vi "sv_Check for Bandwidth Change.vi"(7 "reset filter (F)":bool, 8 "error in (no error)":errorcluster, 9 "1/n octave settings":T2) -> (0 "error out":errorcluster, 1 "bandwidth":T3(ring), 2 "parameter has changed":bool)   [LabVIEW 2017, in "SoundVib_Octave_2014 standard.lvlib"]
uses:
  <vilib>/addons/Sound and Vibration/svt_Octave/SoundVib_Octave_2014 standard.lvlib
  <vilib>/addons/_NISVFA/_Shared subVIs/Controls/svc_Octave Standard.ctl
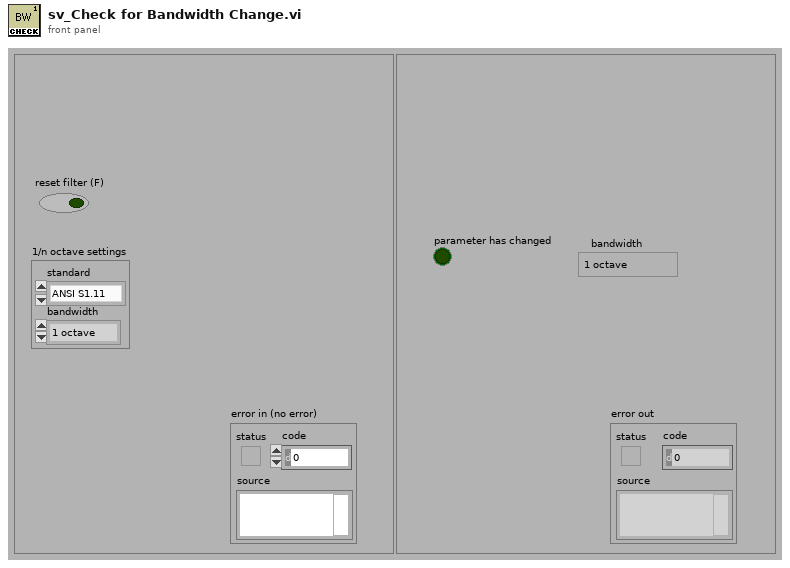
[diagram p1: front panel]
types:
  T1 = typedef "svc_Octave Standard.ctl" = enum16{"ANSI S1.11", "IEC 61260"}
  T2 = cluster{"standard":T1, "bandwidth":enum16{"1 octave", "1/3 octave", "1/6 octave", "1/12 octave", "1/24 octave"}}
  T3 = enum16{"1 octave", "1/3 octave", "1/6 octave", "1/12 octave", "1/24 octave"}
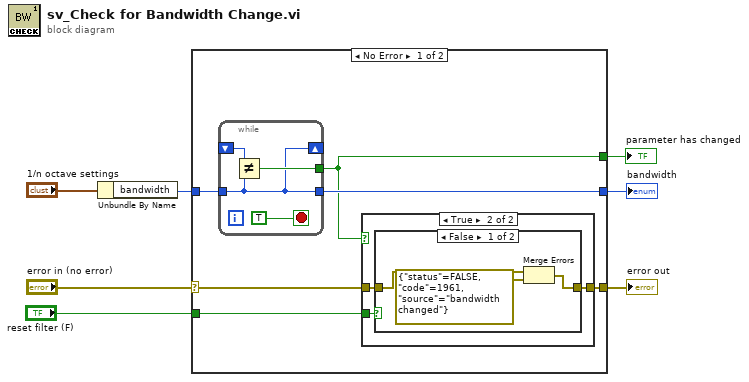
[diagram p0: block diagram]
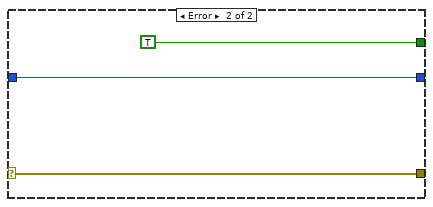
[diagram p4: hidden frame]
diagram:
  n1 = Unbundle By Name("1/n octave settings") -> ("bandwidth"=w4:T3)
  n2 = case shown="No Error" "error in (no error)" {
    selector: "error in (no error)" -> [w10 w28]
    tunnel: [w13 w27] -> w6
    tunnel: [w9 w28] -> w5
    tunnel: w4 -> [w12 w27]
    tunnel: [w11 TRUE] -> w3
    tunnel: "reset filter (F)" -> [w8 _]
    frame No Error {
      n3 = while {
        tunnel: [w14] -> w13
        tunnel: [w16] -> w11
        tunnel: w12 -> [w14]
        shift-left: _ -> [w15]
        shift-right: [w14] -> _
        stop <- TRUE stop-if-true
        n4 = Not Equal?(x=w15, y=w14) -> (x != y?=w16:bool)
      }
      n5 = case shown="True" w11 {
        tunnel: w10 -> [w18 w19]
        tunnel: [w18 w21] -> w9
        tunnel: w8 -> [_ w20]
        frame False {
        }
        frame True {
          n6 = case shown="False" w20 {
            tunnel: [w23 w25] -> w21
            tunnel: w19 -> [w22 w25]
            frame False {
              n7 = Merge Errors(w22, errorcluster {"status"=FALSE, "code"=1961, "source"="bandwidth changed"} ("error IO")) -> (w23:errorcluster)
            }
            frame True {
            }
          }
        }
      }
    }
    frame Error {
    }
  }
  "error out" <- w5
  "bandwidth" <- w6
  "parameter has changed" <- w3
